vi "LJUD UE9RAW FeedbackAlt.vi"(5 "Comm Settings":T1={"Open LabJack "=TRUE, "Use USB"=TRUE, "IP Address"="192.168.1.209", "PortA"=52360, "PortB"=0}, 6 "Digital IN":T4, 8 "error in (no error)":errorcluster, 9 "Analog Outputs":T2={"DAC0"=0, "DAC1"=0, "Update DACs"=TRUE}, 10 "AIN Options":T5={"AINMask"=1, "AIN14Select"=128, "AIN15Select"=136, "ResolutionIndex"=12, "Settling Index"=0, "Bip/Gain (per CH)"=[8, 8, 8, 8, 8, 8, 8, 8, 8, 8, 8, 8, 8, 8, 8, 8], "CH0-CH13 Select"=[0, 1, 2, 3, 4, 5, 6, 7, 8, 9, 10, 11, 12, 13]}, 11 "Handle In":i32) -> (0 "error out":errorcluster, 2 "Analog Inputs":u16[](array[numeric]), 3 "Handle Out":i32, 4 "Digital Out":T3)   [LabVIEW 2021]
panel:
  out "milliseconds":u32
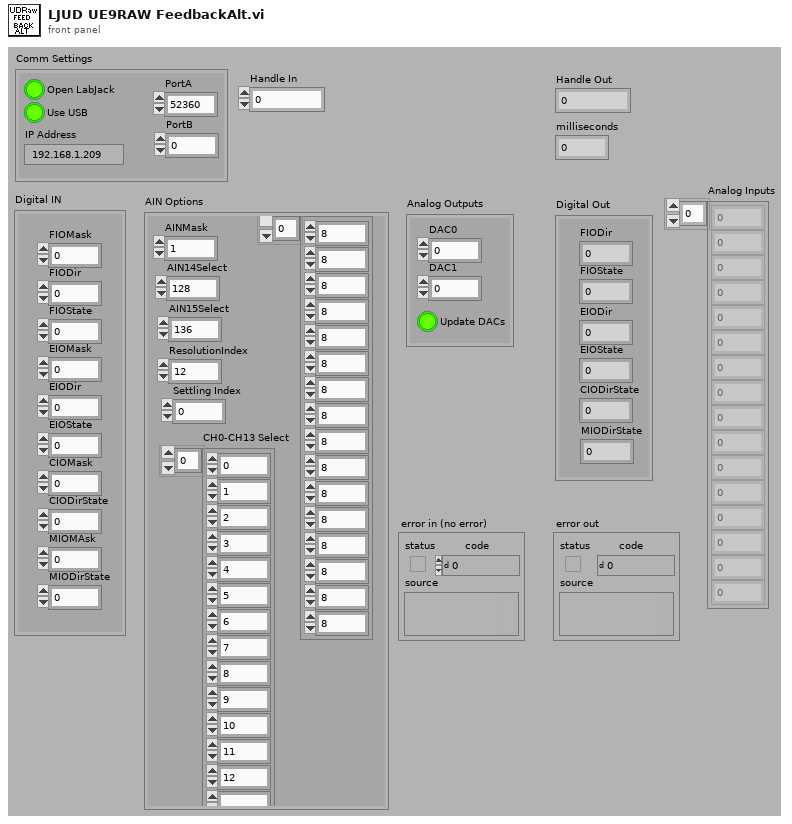
[diagram p1: front panel]
types:
  T1 = cluster{"Open LabJack ":bool, "Use USB":bool, "IP Address":string, "PortA":u16, "PortB":u16}
  T2 = cluster{"DAC0":u16, "DAC1":u16, "Update DACs":bool}
  T3 = cluster{"FIODir":u8, "FIOState":u8, "EIODir":u8, "EIOState":u8, "CIODirState":u8, "MIODirState":u8}
  T4 = cluster{"FIOMask":u8, "FIODir":u8, "FIOState":u8, "EIOMask":u8, "EIODir":u8, "EIOState":u8, "CIOMask":u8, "CIODirState":u8, "MIOMAsk":u8, "MIODirState":u8}
  T5 = cluster{"AINMask":u16, "AIN14Select":u8, "AIN15Select":u8, "ResolutionIndex":u8, "Settling Index":u8, "Bip/Gain (per CH)":u8[], "CH0-CH13 Select":u8[]}
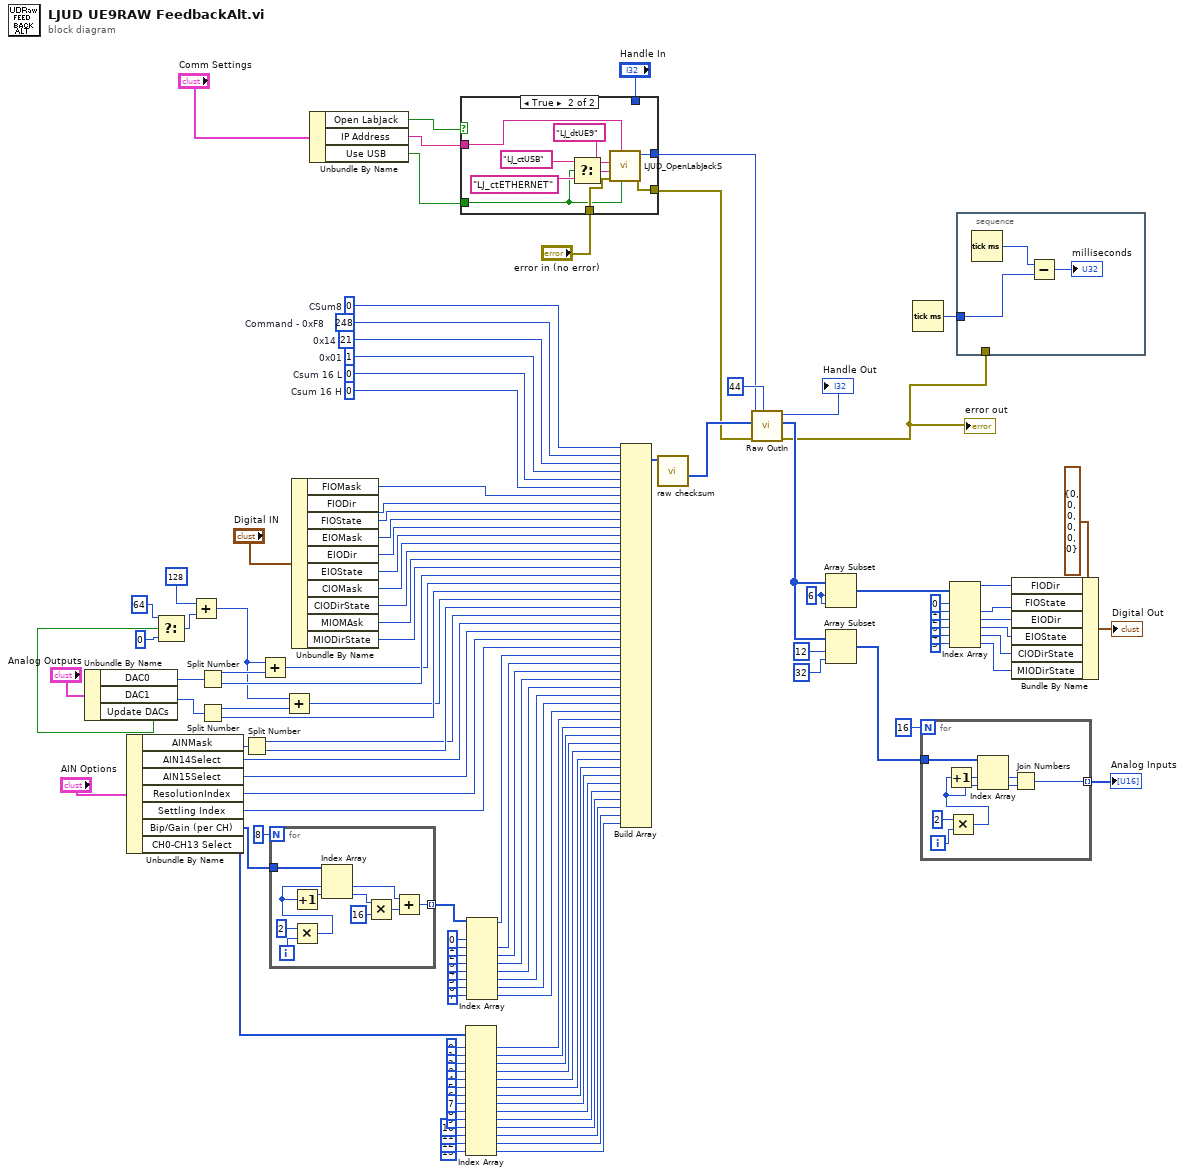
[diagram p0: block diagram]
diagram:
  w85 = 6 ("Array Index")
  w118 = u8 0  # Csum 16 H
  w119 = u8 0  # Csum 16 L
  w120 = u8 1  # 0x01
  w121 = u8 21  # 0x14
  w122 = u8 0  # CSum8
  w124 = u8 248  # Command - 0xF8
  n1 = Unbundle By Name("Analog Outputs") -> ("DAC0"=w104:u16, "DAC1"=w103:u16, "Update DACs"=w42:bool)
  n2 = Unbundle By Name("AIN Options") -> ("AINMask"=w100:u16, "AIN14Select"=w97:u8, "AIN15Select"=w96:u8, "ResolutionIndex"=w95:u8, "Settling Index"=w94:u8, "Bip/Gain (per CH)"=w65:u8[], "CH0-CH13 Select"=w28:u8[])
  n3 = Select(t=u8 64 ("x"), s=w42, f=u8 0 ("x")) -> (s? t:f=w47:u8)
  n4 = Add(x=u8 128, y=w47) -> (x+y=w43:u8)
  n5 = Split Number(x=w104) -> (hi(x)=w53:u8, lo(x)=w102:u8)
  n6 = Split Number(x=w103) -> (hi(x)=w51:u8, lo(x)=w101:u8)
  n7 = Split Number(x=w100) -> (hi(x)=w98:u8, lo(x)=w99:u8)
  n8 = Add(x=w43, y=w53) -> (x+y=w52:u8)
  n9 = for {
    N: 8 -> [_]
    tunnel: w65 -> [w133]
    tunnel: [w125] -> w63 mode=indexing
    i -> [w132]
    n10 = Multiply(x=2, y=w132) -> (x*y=w129:i32)
    n11 = Increment(x=w129) -> (x+1=w128:i32)
    n12 = Index Array(array=w133, index #1=w129, index #2=w128) -> (element #1=w127:u8, element #2=w126:u8)
    n13 = Multiply(x=w126, y=16) -> (x*y=w130:i32)
    n14 = Add(x=w127, y=w130) -> (x+y=w125:i32)
  }
  n15 = Add(x=w43, y=w51) -> (x+y=w50:u8)
  n16 = Unbundle By Name("Digital IN") -> ("FIOMask"=w116:u8, "FIODir"=w115:u8, "FIOState"=w114:u8, "EIOMask"=w113:u8, "EIODir"=w112:u8, "EIOState"=w111:u8, "CIOMask"=w110:u8, "CIODirState"=w109:u8, "MIOMAsk"=w108:u8, "MIODirState"=w107:u8)
  n17 = Unbundle By Name("Comm Settings") -> ("Open LabJack"=w7:bool, "IP Address"=w6:string, "Use USB"=w5:bool)
  n18 = case shown="True" w7 {
    tunnel: w6 -> [_ w139]
    tunnel: "error in (no error)" -> [w136 w143]
    tunnel: [w136 w142] -> w3
    tunnel: [w135 w140] -> w2
    tunnel: w5 -> [_ w141]
    tunnel: "Handle In" -> [w135 _]
    frame False {
    }
    frame True {
      n19 = Select(t="LJ_ctUSB" ("ConnectionType"), s=w141, f="LJ_ctETHERNET" ("ConnectionType")) -> (s? t:f=w137:string)
      n20 = call "LJUD_OpenLabJackS.vi"("FirstFound"=w141, "Address"=w139, "error in"=w143, "ConnectionType"=w137, "DeviceType"="LJ_dtUE9") -> ("error out"=w142:errorcluster, "Handle"=w140:i32)  [unwired: 4 in, 1 out]
    }
  }
  n21 = Index Array(array=w28, index #1=0 ("Index"), index #2=1 ("Index"), index #3=2 ("Index"), index #4=3 ("Index"), index #5=4 ("Index"), index #6=5 ("Index"), index #7=6 ("Index"), index #8=7 ("Index"), index #9=8 ("Index"), index #10=9 ("Index"), index #11=10 ("Index"), index #12=11 ("Index"), index #13=12 ("Index"), index #14=13 ("Index")) -> (element #1=w21:u8, element #2=w20:u8, element #3=w19:u8, element #4=w18:u8, element #5=w17:u8, element #6=w16:u8, element #7=w15:u8, element #8=w14:u8, element #9=w13:u8, element #10=w12:u8, element #11=w11:u8, element #12=w10:u8, element #13=w9:u8, element #14=w8:u8)
  n22 = Index Array(array=w63, index #1=0 ("Index"), index #2=1 ("Index"), index #3=2 ("Index"), index #4=3 ("Index"), index #5=4 ("Index"), index #6=5 ("Index"), index #7=6 ("Index"), index #8=7 ("Index")) -> (element #1=w62:i32, element #2=w61:i32, element #3=w60:i32, element #4=w59:i32, element #5=w58:i32, element #6=w57:i32, element #7=w56:i32, element #8=w55:i32)
  n23 = Build Array(w122, w124, w121, w120, w119, w118, w116, w115, w114, w113, w112, w111, w110, w109, w108, w107, w102, w52, w101, w50, w99, w98, w97, w96, w95, w94, w62, w61, w60, w59, w58, w57, w56, w55, w21, w20, w19, w18, w17, w16, w15, w14, w13, w12, w11, w10, w9, w8) -> (w123:i32[])
  n24 = call "raw checksum.vi"("Array"=w123) -> ("Array Output"=w41:u8[])  [unwired: 3 in, 7 out]
  n25 = call "Raw OutIn.vi"("# of bytes to read in"=44 ("# of bytes to read"), "error in"=w3, "Raw Out"=w41, "Handle In"=w2) -> ("error out"=w37:errorcluster, "Raw In"=w40:u8[], "Handle Out"=→"Handle Out":i32)  [unwired: 4 in, 1 out]
  "error out" <- w37
  n26 = Array Subset(array=w40, index=w85, length=w85) -> (w82:u8[])
  n27 = Array Subset(array=w40, index=12 ("Array Index"), length=32 ("Array Length")) -> (w69:u8[])
  n28 = Tick Count (ms)() -> (millisecond timer value=w49:u32)
  n29 = for {
    N: 16 -> [_]
    tunnel: w69 -> [w151]
    tunnel: [w146] -> w48 mode=indexing
    i -> [w153]
    n30 = Multiply(x=2, y=w153) -> (x*y=w149:i32)
    n31 = Increment(x=w149) -> (x+1=w150:i32)
    n32 = Index Array(array=w151, index #1=w150, index #2=w149) -> (element #1=w148:u8, element #2=w147:u8)
    n33 = Join Numbers(hi=w148, lo=w147) -> ((hi.lo)=w146:u16)
  }
  "Analog Inputs" <- w48
  n34 = Index Array(array=w82, index #1=0 ("Index"), index #2=1 ("Index"), index #3=2 ("Index"), index #4=3 ("Index"), index #5=4 ("Index"), index #6=5 ("Index")) -> (element #1=w75:u8, element #2=w74:u8, element #3=w73:u8, element #4=w72:u8, element #5=w71:u8, element #6=w70:u8)
  n35 = stacked-sequence {
    tunnel: w49 -> [w156]
    tunnel: w37 -> [_]
    frame #0 {
      n36 = Tick Count (ms)() -> (millisecond timer value=w155:u32)
      n37 = Subtract(x=w155, y=w156) -> (x-y=→"milliseconds":u32)
    }
  }
  n38 = Bundle By Name(cluster=T3 {"FIODir"=0, "FIOState"=0, "EIODir"=0, "EIOState"=0, "CIODirState"=0, "MIODirState"=0} ("Digital Out"), "FIODir"=w75, "FIOState"=w74, "EIODir"=w73, "EIOState"=w72, "CIODirState"=w71, "MIODirState"=w70) -> (→"Digital Out":T3)
